vi "Should Stop.vi"(11 "Application Command.lvclass":refnum<class "Application Command.lvclass">) -> (2 "stop?":bool)   [LabVIEW 2010, in "Application Command.lvclass"]
doc: "This method determines whether or not the consumer loop of TLC Main should be halted. This method has a FALSE constant wired to the stop? output. \n\nThis will only be overwritten by the Should Stop method Exit App.lvclass. Any other application function that will always stop execution of the consumer loop would also need to overwrite this method."
uses:
  Application Command.lvclass
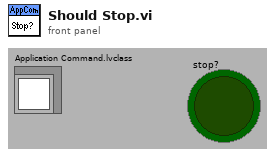
[diagram p1: front panel]
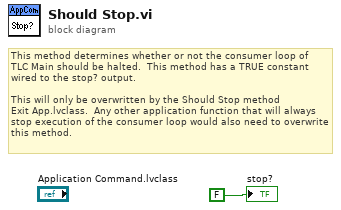
[diagram p0: block diagram]
diagram:
  # "This method determines whether or not the consumer loop of \nTLC Main should be halted.  This method has a TRUE constant \nwired to the stop? output.  \n\nThis will only be overwritten by the Should Stop method \nExit App.lvclass.  Any other application function that will always \nstop execution of the consumer loop would also need to overwrite \nthis method."
  "stop?" <- FALSE ("stop?")
